vi "Configure Trigger (Pattern).vi"(0 "VISA resource name":refnum<visa-resource-name>, 1 "Logic Setting (False)":bool, 2 "Trigger Condition (0:False)":u16(ring) items=["False", "Less Than", "More Than", "True"], 3 "Time (500E-12)":dbl=5e-10, 5 "Channel1 Input":T4={"Channel1 Logic Iput (0:High)"=0, "Channel1 Threshold (1.0v)"=1.0} {"Channel1 Logic Iput (0:High)" items=["High", "Low", "X"]}, 7 "Channel2 Input":T3={"Channel2 Logical Input (0:High) "=0, "Channel2 Threshold (1.0v) "=1.0} {"Channel2 Logical Input (0:High)" items=["High", "Low", "X"]}, 9 "Pattern Type (0:AND)":u16(ring) items=["AND", "NAND", "OR", "NOR"], 11 "error in (no error)":errorcluster, 12 "Channel3 Input":T2={"Channel3 Logical Input (0:High)"=0, "Channel3 Threshold (1.0v)"=1.0} {"Channel3 Logical Input (0:High)" items=["High", "Low", "X"]}, 13 "Channel4 Input":T1={"Channel4 Logical Input (0:High)"=0, "Channel4 Threshold (1.0v)  "=1.0} {"Channel4 Logical Input (0:High)" items=["High", "Low", "X"]}, 14 "Trigger Event (0:A Event)":u16(ring) items=["A Event", "B Event"]) -> (4 "VISA resource name out":refnum<visa-resource-name>, 15 "error out":errorcluster)   [LabVIEW 2011, in "Tektronix 7000 Series.lvlib"]
doc: "Configures Pattern trigger settings for an oscilloscope.Pattern trigger occurs when the specified logical combinations of channels 1, 2, 3, and 4 are met for 4 channels. For 2 channels, pattern trigger occurs when the specified logical combinations of channels 1 and 2 are met. You also can use this Vi to configure the logic patterns.\n\nTDS5000,TDS5000B,TDS6000,CSA7000 and TDS7000 series oscilloscopes don't support B Pattern Trigger."
uses:
  Tektronix 7000 Series.lvlib
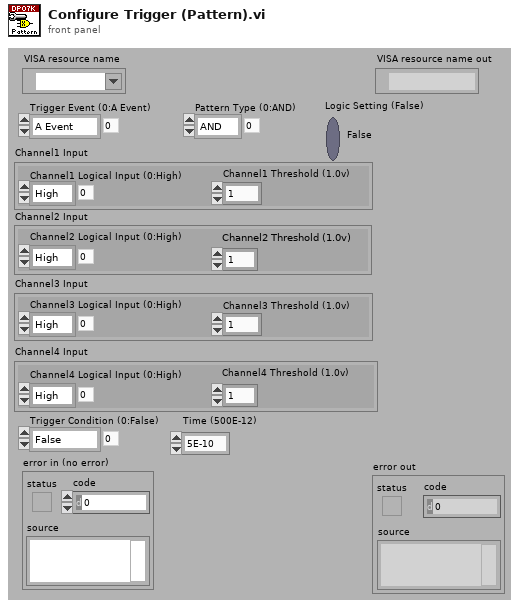
[diagram p1: front panel]
types:
  T1 = cluster{"Channel4 Logical Input (0:High)":u16, "Channel4 Threshold (1.0v)  ":dbl}
  T2 = cluster{"Channel3 Logical Input (0:High)":u16, "Channel3 Threshold (1.0v)":dbl}
  T3 = cluster{"Channel2 Logical Input (0:High) ":u16, "Channel2 Threshold (1.0v) ":dbl}
  T4 = cluster{"Channel1 Logic Iput (0:High)":u16, "Channel1 Threshold (1.0v)":dbl}
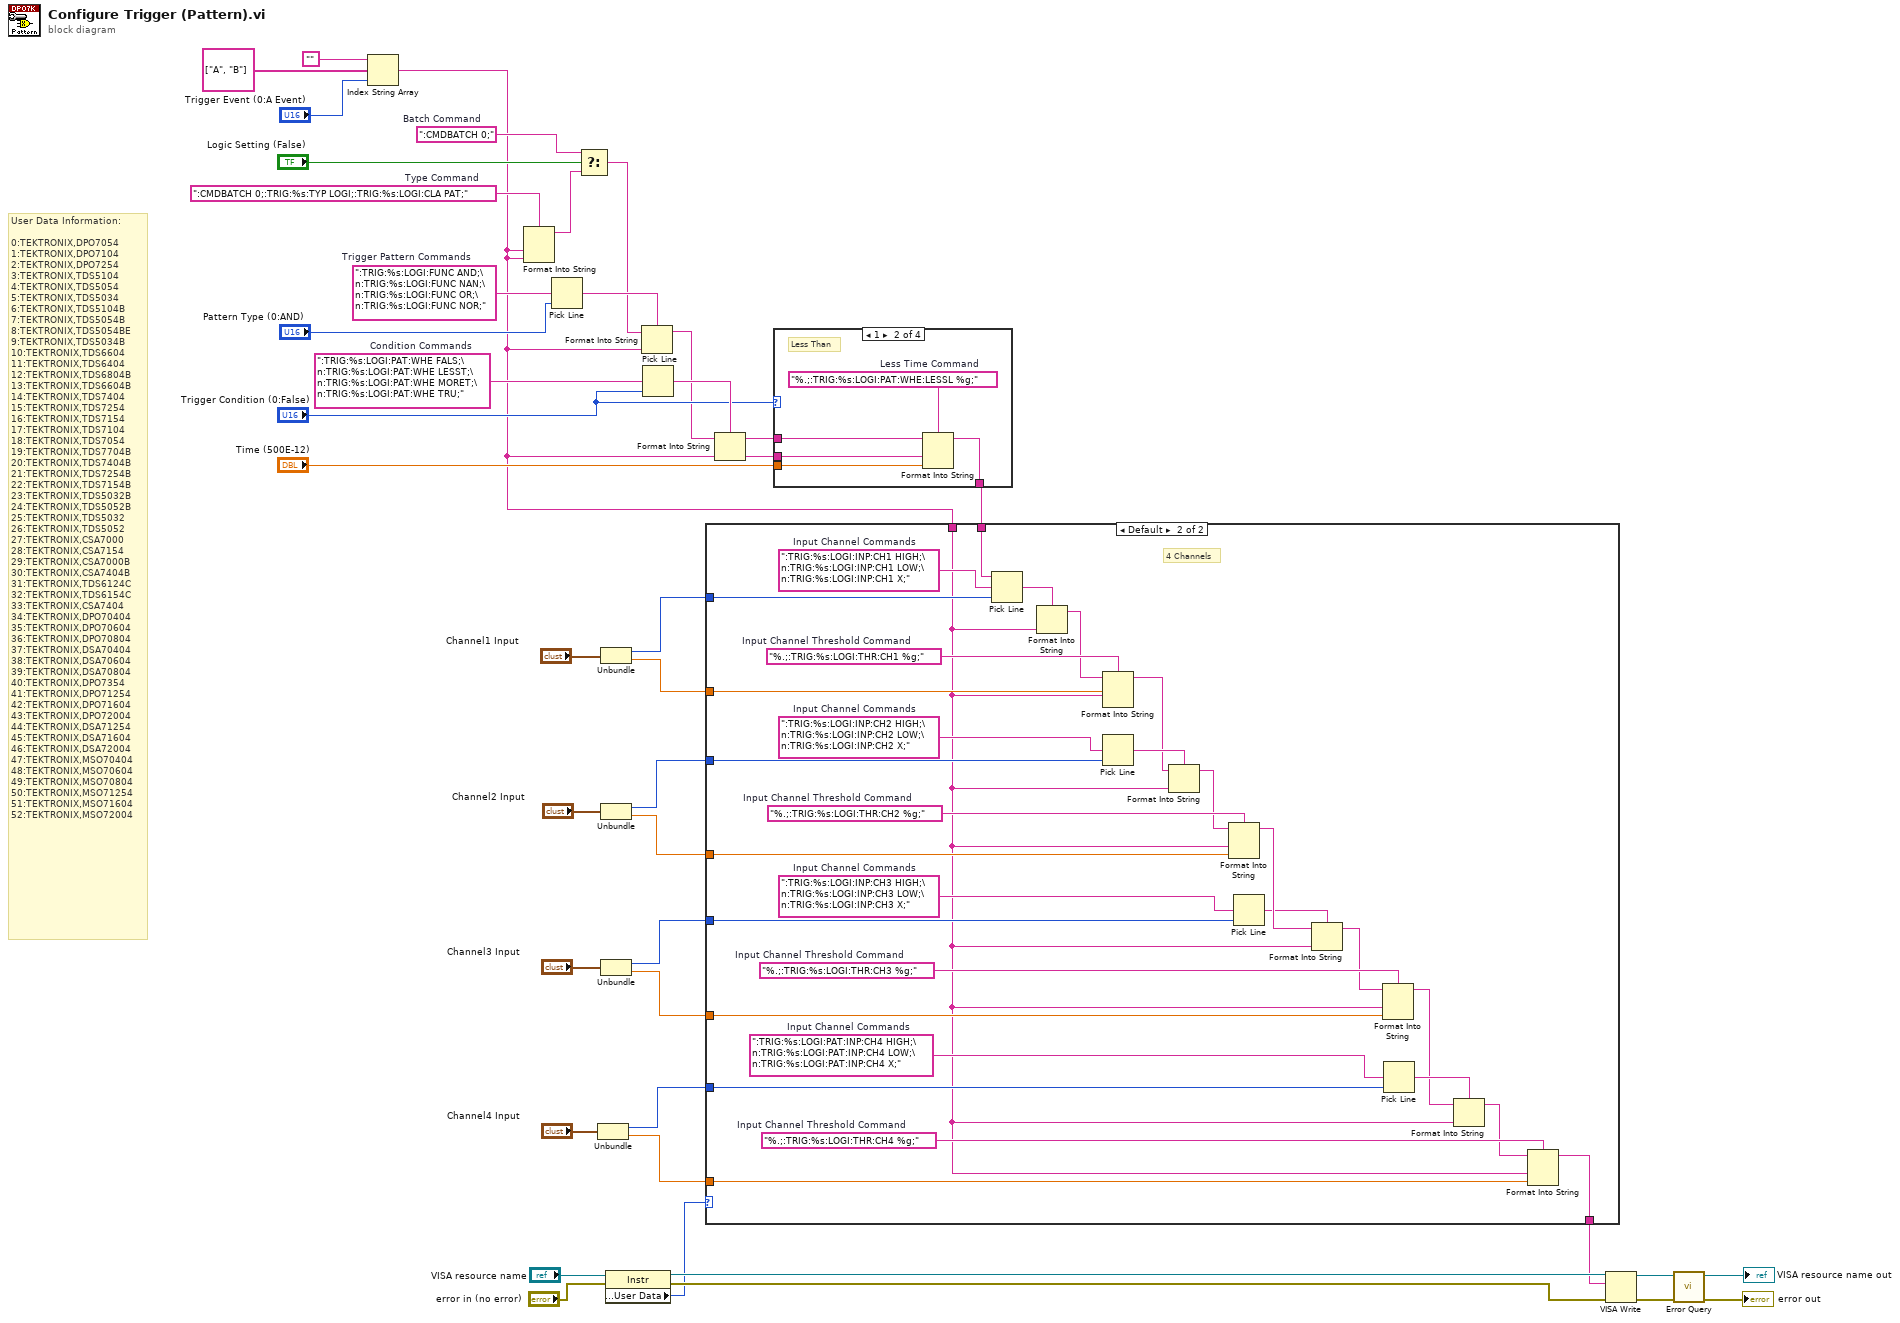
[diagram p0: block diagram]
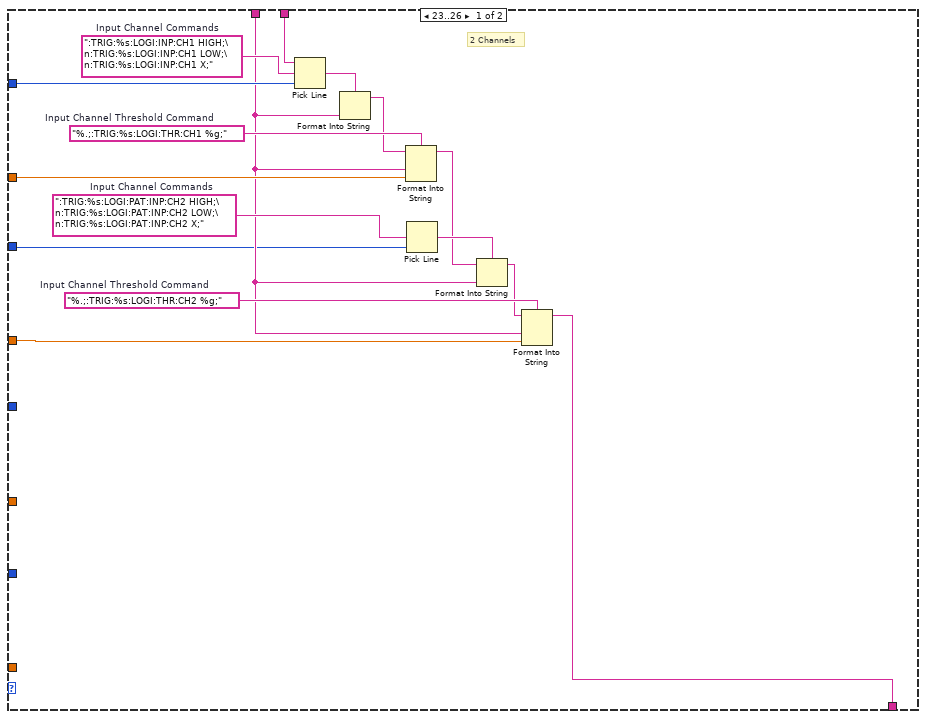
[diagram p2: hidden frame]
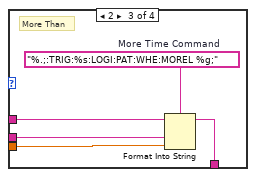
[diagram p4: hidden frame]
diagram:
  w23 = ":CMDBATCH 0;:TRIG:%s:TYP LOGI;:TRIG:%s:LOGI:CLA PAT;"  # Type Command
  w26 = ":TRIG:%s:LOGI:PAT:WHE FALS;\n:TRIG:%s:LOGI:PAT:WHE LESST;\n:TRIG:%s:LOGI:PAT:WHE MORET;\n:TRIG:%s:LOGI:PAT:WHE TRU;"  # Condition Commands
  w27 = ":TRIG:%s:LOGI:FUNC AND;\n:TRIG:%s:LOGI:FUNC NAN;\n:TRIG:%s:LOGI:FUNC OR;\n:TRIG:%s:LOGI:FUNC NOR;"  # Trigger Pattern Commands
  w25 = ":CMDBATCH 0;"  # Batch Command
  # "User Data Information:\n\n0:TEKTRONIX,DPO7054\n1:TEKTRONIX,DPO7104\n2:TEKTRONIX,DPO7254\n3:TEKTRONIX,TDS5104\n4:TEKTRONIX,TDS5054\n5:TEKTRONIX,TDS5034\n6:TEKTRONIX,TDS5104B\n7:TEKTRONIX,TDS5054B\n8:TEKTRONIX,TDS5054BE\n9:TEKTRONIX,TDS5034B\n10:TEKTRONIX,TDS6604\n11:TEKTRONIX,TDS6404\n12:TEKTRONIX,TDS6804B\n13:TEKTRONIX,TDS6604B\n14:TEKTRONIX,TDS7404\n15:TEKTRONIX,TDS7254\n16:TEKTRONIX,TDS7154\n17:TEKTRONIX,TDS7104\n18:TEKTRONIX,TDS7054\n19:TEKTRONIX,TDS7704B\n20:TEKTRONIX,TDS7404B\n21:TEKTRONIX,TDS7254B\n22:TEKTRONIX,TDS7154B\n23:TEKTRONIX,TDS5032B\n24:TEKTRONIX,TDS5052B\n25:TEKTRONIX,TDS5032\n26:TEKTRONIX,TDS5052\n27:TEKTRONIX,CSA7000\n28:TEKTRONIX,CSA7154\n29:TEKTRONIX,CSA7000B\n30:TEKTRONIX,CSA7404B\n31:TEKTRONIX,TDS6124C\n32:TEKTRONIX,TDS6154C\n33:TEKTRONIX,CSA7404\n34:TEKTRONIX,DPO70404\n35:TEKTRONIX,DPO70604\n36:TEKTRONIX,DPO70804\n37:TEKTRONIX,DSA70404\n38:TEKTRONIX,DSA70604\n39:TEKTRONIX,DSA70804\n40:TEKTRONIX,DPO7354\n41:TEKTRONIX,DPO71254\n42:TEKTRONIX,DPO71604\n43:TEKTRONIX,DPO72004\n44:TEKTRONIX,DSA71254\n45:TEKTRONIX,DSA71604\n46:TEKTRONIX,DSA72004\n47:TEKTRONIX,MSO70404\n48:TEKTRONIX,MSO70604\n49:TEKTRONIX,MSO70804\n50:TEKTRONIX,MSO71254\n51:TEKTRONIX,MSO71604\n52:TEKTRONIX,MSO72004"
  n1 = Index String Array(1:"Trigger Event (0:A Event)", 2:string[] ["A", "B"], 3:"" ("Empty String Constant")) -> (0:w5:string)
  n2 = Format Into String(format string=w23, w5, w5) -> (resulting string=w22:string)  [unwired: 2 in, 1 out]
  n3 = Pick Line(multi-line string=w27, line index="Pattern Type (0:AND)") -> (output string=w21:string)  [unwired: 1 in]
  n4 = Select(t=w25, s="Logic Setting (False)", f=w22) -> (s? t:f=w20:string)
  n5 = Unbundle("Channel4 Input") -> ("Channel4 Logical Input (0:High)"=w35:u16, "Channel4 Threshold (1.0v)"=w16:dbl)
  n6 = Unbundle("Channel1 Input") -> ("Channel1 Logic Iput (0:High)"=w39:u16, "Channel1 Threshold (1.0v)"=w12:dbl)
  n7 = Unbundle("Channel2 Input") -> ("Channel2 Logical Input (0:High)"=w19:u16, "Channel2 Threshold (1.0v)"=w18:dbl)
  n8 = Unbundle("Channel3 Input") -> ("Channel3 Logical Input (0:High)"=w2:u16, "Channel3 Threshold (1.0v)"=w17:dbl)
  n9 = property class="Instr"(reference="VISA resource name", error in="error in (no error)") -> (reference out=w8:refnum<visa-resource-name>, error out=w6:errorcluster, "General Settings:User Data"=w3:u32)
  n10 = Format Into String(format string=w21, initial string=w20, w5) -> (resulting string=w10:string)  [unwired: 1 in, 1 out]
  n11 = Pick Line(multi-line string=w26, line index="Trigger Condition (0:False)") -> (output string=w15:string)  [unwired: 1 in]
  n12 = Format Into String(format string=w15, initial string=w10, w5) -> (resulting string=w14:string)  [unwired: 1 in, 1 out]
  n13 = case shown="1" "Trigger Condition (0:False)" {
    tunnel: w14 -> [w42 w47 w51 w53]
    tunnel: [w42 w45 w50 w53] -> w4
    tunnel: w5 -> [_ w43 w49 _]
    tunnel: "Time (500E-12)" -> [_ w44 w48 _]
    frame 0, Default {
      # "False"
    }
    frame 1 {
      w46 = "%.;:TRIG:%s:LOGI:PAT:WHE:LESSL %g;"  # Less Time Command
      # "Less Than"
      n14 = Format Into String(format string=w46, initial string=w47, w43, w44) -> (resulting string=w45:string)  [unwired: 1 in, 1 out]
    }
    frame 2 {
      w52 = "%.;:TRIG:%s:LOGI:PAT:WHE:MOREL %g;"  # More Time Command
      # "More Than"
      n15 = Format Into String(format string=w52, initial string=w51, w49, w48) -> (resulting string=w50:string)  [unwired: 1 in, 1 out]
    }
    frame 3 {
      # "True"
    }
  }
  n16 = case shown="Default" w3 {
    tunnel: w39 -> [w65 w99]
    tunnel: w2 -> [_ w98]
    tunnel: w35 -> [_ w97]
    tunnel: w19 -> [w56 w86]
    tunnel: w18 -> [w55 w83]
    tunnel: w17 -> [_ w78]
    tunnel: w16 -> [_ w75]
    tunnel: w12 -> [w64 w73]
    tunnel: w5 -> [w58 w72]
    tunnel: w4 -> [w63 w71]
    tunnel: [w54 w70] -> w1
    frame 23..26 {
      w62 = "%.;:TRIG:%s:LOGI:THR:CH2 %g;"  # Input Channel Threshold Command
      w61 = ":TRIG:%s:LOGI:PAT:INP:CH2 HIGH;\n:TRIG:%s:LOGI:PAT:INP:CH2 LOW;\n:TRIG:%s:LOGI:PAT:INP:CH2 X;"  # Input Channel Commands
      w68 = "%.;:TRIG:%s:LOGI:THR:CH1 %g;"  # Input Channel Threshold Command
      w69 = ":TRIG:%s:LOGI:INP:CH1 HIGH;\n:TRIG:%s:LOGI:INP:CH1 LOW;\n:TRIG:%s:LOGI:INP:CH1 X;"  # Input Channel Commands
      # "2 Channels"
      n17 = Pick Line(string ("")=w63, multi-line string=w69, line index=w65) -> (output string=w67:string)
      n18 = Format Into String(format string=w67, w58) -> (resulting string=w66:string)  [unwired: 2 in, 1 out]
      n19 = Format Into String(format string=w68, initial string=w66, w58, w64) -> (resulting string=w57:string)  [unwired: 1 in, 1 out]
      n20 = Pick Line(multi-line string=w61, line index=w56) -> (output string=w60:string)  [unwired: 1 in]
      n21 = Format Into String(format string=w60, initial string=w57, w58) -> (resulting string=w59:string)  [unwired: 1 in, 1 out]
      n22 = Format Into String(format string=w62, initial string=w59, w58, w55) -> (resulting string=w54:string)  [unwired: 1 in, 1 out]
    }
    frame Default {
      w90 = "%.;:TRIG:%s:LOGI:THR:CH4 %g;"  # Input Channel Threshold Command
      w89 = ":TRIG:%s:LOGI:PAT:INP:CH4 HIGH;\n:TRIG:%s:LOGI:PAT:INP:CH4 LOW;\n:TRIG:%s:LOGI:PAT:INP:CH4 X;"  # Input Channel Commands
      w91 = "%.;:TRIG:%s:LOGI:THR:CH3 %g;"  # Input Channel Threshold Command
      w92 = ":TRIG:%s:LOGI:INP:CH3 HIGH;\n:TRIG:%s:LOGI:INP:CH3 LOW;\n:TRIG:%s:LOGI:INP:CH3 X;"  # Input Channel Commands
      w94 = "%.;:TRIG:%s:LOGI:THR:CH2 %g;"  # Input Channel Threshold Command
      w93 = ":TRIG:%s:LOGI:INP:CH2 HIGH;\n:TRIG:%s:LOGI:INP:CH2 LOW;\n:TRIG:%s:LOGI:INP:CH2 X;"  # Input Channel Commands
      w95 = "%.;:TRIG:%s:LOGI:THR:CH1 %g;"  # Input Channel Threshold Command
      w96 = ":TRIG:%s:LOGI:INP:CH1 HIGH;\n:TRIG:%s:LOGI:INP:CH1 LOW;\n:TRIG:%s:LOGI:INP:CH1 X;"  # Input Channel Commands
      # "4 Channels"
      n23 = Pick Line(string ("")=w71, multi-line string=w96, line index=w99) -> (output string=w88:string)
      n24 = Format Into String(format string=w88, w72) -> (resulting string=w87:string)  [unwired: 2 in, 1 out]
      n25 = Format Into String(format string=w95, initial string=w87, w72, w73) -> (resulting string=w84:string)  [unwired: 1 in, 1 out]
      n26 = Pick Line(multi-line string=w93, line index=w86) -> (output string=w85:string)  [unwired: 1 in]
      n27 = Format Into String(format string=w85, initial string=w84, w72) -> (resulting string=w82:string)  [unwired: 1 in, 1 out]
      n28 = Format Into String(format string=w94, initial string=w82, w72, w83) -> (resulting string=w81:string)  [unwired: 1 in, 1 out]
      n29 = Pick Line(multi-line string=w92, line index=w98) -> (output string=w80:string)  [unwired: 1 in]
      n30 = Format Into String(format string=w80, initial string=w81, w72) -> (resulting string=w79:string)  [unwired: 1 in, 1 out]
      n31 = Format Into String(format string=w91, initial string=w79, w72, w78) -> (resulting string=w76:string)  [unwired: 1 in, 1 out]
      n32 = Pick Line(multi-line string=w89, line index=w97) -> (output string=w77:string)  [unwired: 1 in]
      n33 = Format Into String(format string=w77, initial string=w76, w72) -> (resulting string=w74:string)  [unwired: 1 in, 1 out]
      n34 = Format Into String(format string=w90, initial string=w74, w72, w75) -> (resulting string=w70:string)  [unwired: 1 in, 1 out]
    }
  }
  n35 = VISA Write(VISA resource name=w8, write buffer=w1, error in (no error)=w6) -> (VISA resource name out=w34:refnum<visa-resource-name>, error out=w33:errorcluster)  [unwired: 1 out]
  n36 = call "Error Query.vi"("error in (no error)"=w33, "VISA resource name"=w34) -> ("error out"=→"error out":errorcluster, "VISA resource name out"=→"VISA resource name out":refnum<visa-resource-name>)  [unwired: 6 in, 2 out]
